vi "GetValuesMatchingXPath.vi"(8 "error in (no error)":errorcluster, 10 "XPath":string, 11 "XML refnum in":refnum<k20>) -> (0 "error out":errorcluster, 2 "Values":string[](array[string]), 3 "XML refnum out":refnum<k20>)   [LabVIEW 2027, in "VeriStandTestUtilities.lvlib"]
uses:
  VeriStandTestUtilities.lvlib
  <vilib>/xml/XPath/Get All Matched Nodes (String).vi
  <vilib>/xml/Close Reference(Node).vi
  <resource>/objmgr/DOMUserDefRef.rc
  <vilib>/xml/NI_XML.lvlib
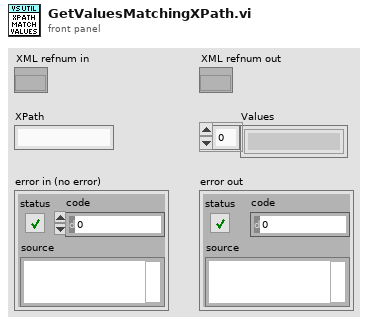
[diagram p1: front panel]
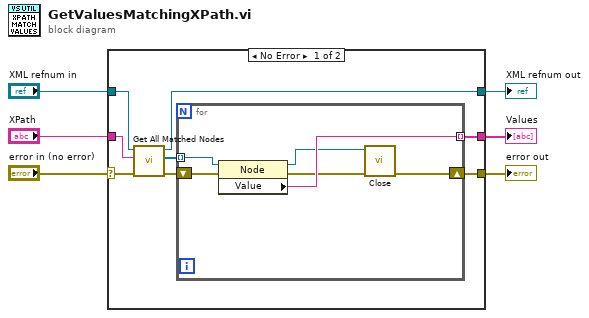
[diagram p0: block diagram]
diagram:
  n1 = case shown="No Error" "error in (no error)" {
    selector: "error in (no error)" -> [w10 w21]
    tunnel: [w14 w21] -> w6
    tunnel: [w13 _] -> w5
    tunnel: "XPath" -> [w12 _]
    tunnel: [w11 w22] -> w3
    tunnel: "XML refnum in" -> [w9 w22]
    frame No Error {
      n2 = call-poly <vilib>:"Get All Matched Nodes.vi"("error in (no error)"=w10, "XPath expression"=w12, "node in"=w9) -> ("error out"=w7:errorcluster, "node result array"=w8:refnum<k20>[], "node out"=w11:refnum<k20>)  [unwired: 6 in]
      n3 = for {
        shift-right: [w16] -> w14
        shift-left: w7 -> [w20]
        tunnel: w8 -> [w19] mode=indexing
        tunnel: [w18] -> w13 mode=indexing
        n4 = property class="Node"(reference=w19, error in=w20) -> (reference out=w15:refnum<k20>, error out=w17:errorcluster, "Value"=w18:string)
        n5 = call-poly <vilib>:"Close.vi"("error in (no error)"=w17, "node"=w15) -> ("error out"=w16:errorcluster)  [unwired: 7 out]
      }
    }
    frame Error {
    }
  }
  "error out" <- w6
  "Values" <- w5
  "XML refnum out" <- w3
